vi "Icon_Convert Height to Rows.vi"(4 "Height":u32) -> (1 "Rows":u32)   [LabVIEW 2009]
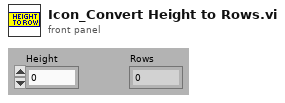
[diagram p1: front panel]
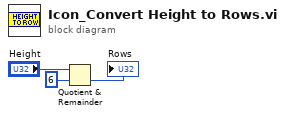
[diagram p0: block diagram]
diagram:
  n1 = Quotient & Remainder(x="Height", y=u32 6) -> (floor(x/y)=→"Rows":u32)  [unwired: 1 out]
